vi "RichToFlatcif_pluginloader_LoadPluginRequest.vi"(5 "OutputClusterType":T1, 11 "InputCluster":T2) -> (3 "OutputCluster":T1)   [LabVIEW 2021, in "CIF_PluginLoader_server.lvlib"]
uses:
  CIF_PluginLoader_server.lvlib
  cif_pluginloader_LoadPluginRequest.ctl
  cif_pluginloader_LoadPluginRequest_Flat.ctl
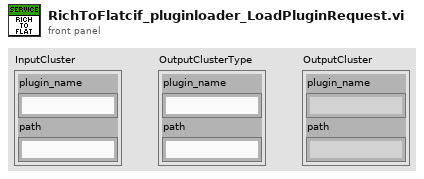
[diagram p1: front panel]
types:
  T1 = typedef "CIF_PluginLoader_server.lvlib/cif_pluginloader_LoadPluginRequest_Flat.ctl" = cluster{"plugin_name":string, "path":string}
  T2 = typedef "CIF_PluginLoader_server.lvlib/cif_pluginloader_LoadPluginRequest.ctl" = cluster{"plugin_name":string, "path":string}
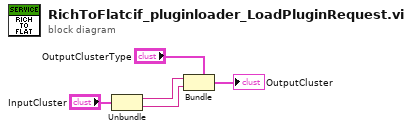
[diagram p0: block diagram]
diagram:
  n1 = Unbundle "Unbundle"("InputCluster") -> ("plugin_name"=w2:string, "path"=w1:string)
  n2 = Bundle "Bundle"(cluster="OutputClusterType", "plugin_name"=w2, "path"=w1) -> (→"OutputCluster":T1)
